vi "Dequeue.vi"(8 "错误输入（无错误）":errorcluster, 11 "MessageQueue":refnum<queue>) -> (0 "错误输出":errorcluster, 1 "Message Data":variant, 2 "Message":string, 3 "MessageQueue":refnum<queue>)   [LabVIEW 2019, in "module.lvlib"]
uses:
  module.lvlib
  Message.ctl
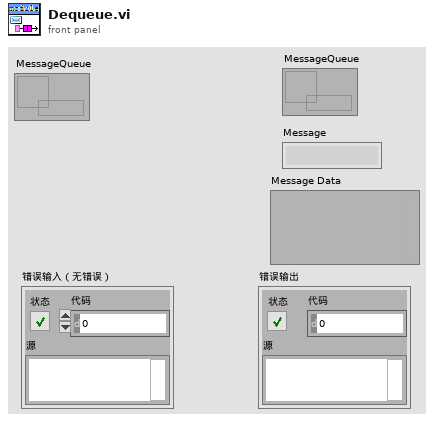
[diagram p1: front panel]
types:
  T1 = typedef "module.lvlib/Message.ctl" = cluster{"Message":string, "Message Data":variant}
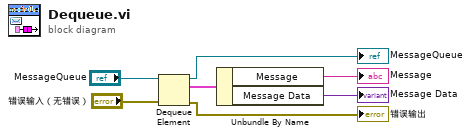
[diagram p0: block diagram]
diagram:
  n1 = Dequeue Element(queue="MessageQueue", error in (no error)="错误输入（无错误）") -> (queue out=→"MessageQueue":refnum<queue>, element=w3:T1, error out=→"错误输出":errorcluster)  [unwired: 1 in, 1 out]
  n2 = Unbundle By Name(w3) -> ("Message"=→"Message":string, "Message Data"=→"Message Data":variant)
